vi "Compute Sum of Gates Plot.vi"(4 "SDV (s)":dbl=160.0, 6 "Gaussian IRF":bool, 8 "Error In":errorcluster, 10 "Phasor Parameters":T1={"Display Parameters"={"# Points"=0, "Ramp Type"=enum."Linear", "Type of Series"=enum."1-Exp Decays", "Min tau"=0.0, "Max tau"=0.0, "Include 0"=FALSE, "Include Infinity"=FALSE}, "Phasor Parameters"={"Harmonic frequency"=0.0, "Use f* = 1/D Frequency"=FALSE, "Calibrated Phasor"=FALSE, "Calibration Lifetime"=1e-09, "Phasor Calculation"=enum."Direct Sum", "SEPL Type"=enum."UC", "# Gates"=1.0, "Square Gate Width"=1e-09, "Show Ticks"=FALSE}, "Decay & IRF Parameters"={"Lifetime"=0.0, "IRF Offset"=0.0, "Laser Period"=0.0, "Normalized Decays"=FALSE, "IRF Model"=enum."Dirac", "IRF Parameter 1"=0.0}, "Gate Parameters"={"First Gate Start"=0.0, "Use Gate Center"=FALSE, "Gate Width"=0.0, "Gate Step"=0.0, "# Gates"=0.0, "Gate Type"=enum."Square", "Edge Width"=0.0, "Top Slope"=0.0, "Reversed Sawtooth?"=FALSE, "Analytical Computation"=FALSE, "Tolerance"=1.0, "Integration"=enum."Item 0", "# Steps"=1.0, "Type of User-defined Function"=enum."Gate"}, "Detector Parameters"={"Frames/Image"=0, "Gates/Frame"=0, "Bits/Frame"=0, "Multiplicity"=0, "Incident Signal"=0.0}} {"Detector Parameters"."Frames/Image" min=1; "Detector Parameters"."Multiplicity" min=0; "Detector Parameters"."Bits/Frame" min=1; "Detector Parameters"."Gates/Frame" min=1; "Gate Parameters"."# Steps" min=0.0; "Gate Parameters"."Tolerance" min=0.0; "Gate Parameters"."Top Slope" min=0.0; "Gate Parameters"."Edge Width" min=0.0; "Gate Parameters"."Gate Step" min=0.0; "Gate Parameters"."# Gates" min=0.0 step=1.0; "Gate Parameters"."Gate Width" min=0.0; "Decay & IRF Parameters"."Lifetime" min=0.0; "Decay & IRF Parameters"."Laser Period" min=0.0; "Phasor Parameters"."Square Gate Width" min=0.0; "Phasor Parameters"."# Gates" min=0.0; "Phasor Parameters"."Calibration Lifetime" min=0.0; "Phasor Parameters"."Harmonic frequency" min=0.0; "Display Parameters"."Min tau" min=0.0; "Display Parameters"."Max tau" min=0.0; "Display Parameters"."# Points" min=1 step=1}, 11 "Sum of Gates Graph Refnum":refnum<vi>) -> (0 "Error Out":errorcluster, 3 "Sum of Gates Plot":cluster{"Array":dbl[], "Array":dbl[]})   [LabVIEW 2019]
uses:
  Pseudo Phasor Parameters.ctl
  Phasor Explorer Display Parameters.ctl
  Type of Series.ctl
  Phasor Explorer Phasor Parameters.ctl
  Phasor Calculation Type.ctl
  Phasor Type.ctl
  Phasor Explorer Decay Parameters.ctl
  IRF Model.ctl
  Phasor Explorer Gate Parameters.ctl
  Gate Type.ctl
  Phasor Explorer Detector Parameters.ctl
  Linear Ramp End Options.ctl
  <vilib>/Utility/error.llb/Error Cluster From Error Code.vi
  SEPXP Globals.vi
  <vilib>/ErrorRing/Error Ring.xnode
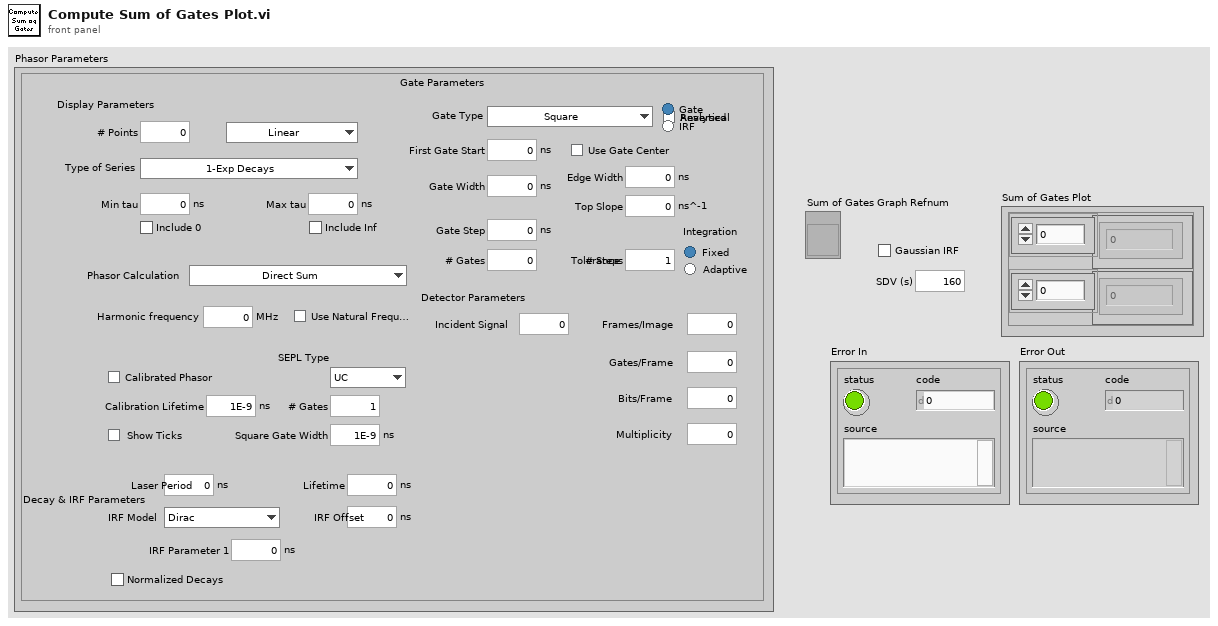
[diagram p1: front panel]
types:
  T1 = typedef "Pseudo Phasor Parameters.ctl" = cluster{"Display Parameters":T2, "Phasor Parameters":T4, "Decay & IRF Parameters":T7, "Gate Parameters":T9, "Detector Parameters":T11}
  T2 = typedef "Phasor Explorer Display Parameters.ctl" = cluster{"# Points":i32, "Ramp Type":enum16{"Linear", "Logarithmic"}, "Type of Series":T3, "Min tau":dbl[unit], "Max tau":dbl[unit], "Include 0":bool, "Include Infinity":bool}
  T3 = typedef "Type of Series.ctl" = enum16{"1-Exp Decays", "Linear Combination of 1-Exp"}
  T4 = typedef "Phasor Explorer Phasor Parameters.ctl" = cluster{"Harmonic frequency":dbl[unit], "Use f* = 1/D Frequency":bool, "Calibrated Phasor":bool, "Calibration Lifetime":dbl[unit], "Phasor Calculation":T5, "SEPL Type":T6, "# Gates":dbl, "Square Gate Width":dbl[unit], "Show Ticks":bool}
  T5 = typedef "Phasor Calculation Type.ctl" = enum16{"Direct Sum", "Analytical Formula"}
  T6 = typedef "Phasor Type.ctl" = enum16{"UC", "L_N", "L_N[W]"}
  T7 = typedef "Phasor Explorer Decay Parameters.ctl" = cluster{"Lifetime":dbl[unit], "IRF Offset":dbl[unit], "Laser Period":dbl[unit], "Normalized Decays":bool, "IRF Model":T8, "IRF Parameter 1":dbl[unit]}
  T8 = typedef "IRF Model.ctl" = enum16{"Dirac", "Exponential"}
  T9 = typedef "Phasor Explorer Gate Parameters.ctl" = cluster{"First Gate Start":dbl[unit], "Use Gate Center":bool, "Gate Width":dbl[unit], "Gate Step":dbl[unit], "# Gates":dbl, "Gate Type":T10, "Edge Width":dbl[unit], "Top Slope":dbl[unit], "Reversed Sawtooth?":bool, "Analytical Computation":bool, "Tolerance":dbl, "Integration":enum32{"Item 0", "Item 1"}, "# Steps":dbl, "Type of User-defined Function":enum32{"Gate", "IRF"}}
  T10 = typedef "Gate Type.ctl" = enum16{"Square", "Finite Edge Square", "Finite Edge, Tilted Top Square", "Triangle", "Sawtooth", "User-defined"}
  T11 = typedef "Phasor Explorer Detector Parameters.ctl" = cluster{"Frames/Image":i32, "Gates/Frame":i32, "Bits/Frame":i32, "Multiplicity":i32, "Incident Signal":dbl}
  T12 = typedef "Linear Ramp End Options.ctl" = enum16{"Include Min/Exclude Max", "Exclude Min/Include Max", "Include Both Ends", "Exclude Both Ends"}
  T13 = typedef "Gate Definitions.ctl" = cluster{"First Gate: t1":ext, "Gate Width: W":ext, "Gate Step: d":ext, "# Gates: G":ext, "Use Gate Center":bool, "Frames/Image: F":i32, "Gates/Frame: L":i32, "Bits/Frame: q":i32, "Multiplicity: p":i32, "Gate Type":T10, "Gate Edge s":ext, "Gate Top Slope":ext, "Reversed Sawtooth?":bool, "Computation":bool, "User-defined Gate":T14, "Tolerance":ext, "Integration":enum32{"Item 0", "Item 1"}, "# Steps":ext, "Type of User-defined Function":enum32{"Gate", "IRF"}}
  T14 = typedef "XY Plot Data.ctl" = cluster{"X Array":dbl[], "Y Array":dbl[]}
  T15 = typedef "Decay Definiton.ctl" = cluster{"offset: t0":ext, "period: T":ext, "lifetime: tau":ext, "Incident Signal: I":ext, "Normalized Decays":bool, "IRF Model":T8, "IRF Parameter 1":ext}
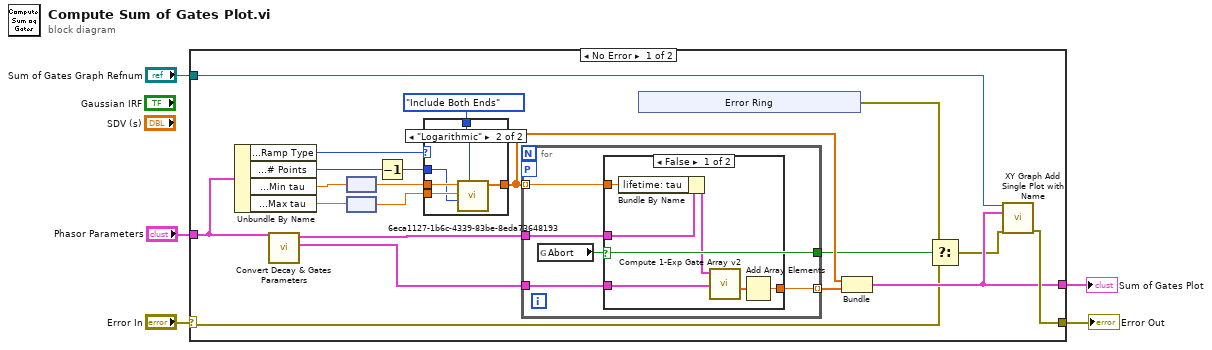
[diagram p0: block diagram]
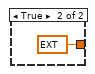
[diagram p2: hidden frame]
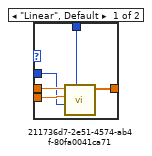
[diagram p3: hidden frame]
diagram:
  n1 = case shown="No Error" "Error In" {
    selector: "Error In" -> [w8 w52]
    tunnel: "Phasor Parameters" -> [w13 _]
    tunnel: "Sum of Gates Graph Refnum" -> [w21 _]
    tunnel: [w20 w52] -> w2
    tunnel: [w14 _] -> w1
    frame No Error {
      n2 = Unbundle By Name(w13) -> ("Display Parameters.Ramp Type"=w19:enum16{"Linear", "Logarithmic"}, "Display Parameters.# Points"=w16:i32, "Display Parameters.Min tau"=w24:dbl[unit], "Display Parameters.Max tau"=w25:dbl[unit])
      n3 = call "Convert Decay & Gates Parameters.vi"("Phasor Parameters"=w13) -> ("Gates Definitions"=w11:T13, "Decay Definition"=w12:T15)  [unwired: 9 in]
      n4 = node(w24) -> (w23:dbl)
      n5 = node(w25) -> (w22:dbl)
      n6 = Decrement(x=w16) -> (x-1=w17:i32)
      n7 = case shown="\"Logarithmic\"" w19 {
        tunnel: w23 -> [w46 w49]
        tunnel: w22 -> [w45 w48]
        tunnel: w17 -> [w44 w47]
        tunnel: [w43 w51] -> w10
        tunnel: Linear_Ramp_End_Options."Include Both Ends" ("Options") -> [w42 w50]
        frame "Linear", Default {
          n8 = call "211736d7-2e51-4574-ab4f-80fa0041ca71.vi"("Options"=w42, "# Steps (1)"=w44, "End (1)"=w45, "Start (0)"=w46) -> ("Ramp"=w43:dbl[])  [unwired: 6 in, 1 out]
        }
        frame "Logarithmic" {
          n9 = call "6eca1127-1b6c-4339-83be-8eda73648193.vi"("Options"=w50, "# Steps (1)"=w47, "End (1)"=w48, "Start (1)"=w49) -> ("Ramp"=w51:dbl[])  [unwired: 6 in, 1 out]
        }
      }
      n10 = for {
        tunnel: w10 -> [w34] mode=indexing
        tunnel: w11 -> [w32]
        tunnel: w12 -> [w33]
        tunnel: [w31] -> w15 mode=indexing
        workers-P: _ -> [_]
        tunnel: [w30] -> w9
        n11 = global read "SEPXP Globals.vi" "Abort"() -> (w30:bool)
        n12 = case shown="False" w30 {
          tunnel: w34 -> [w40 _]
          tunnel: w33 -> [w39 _]
          tunnel: w32 -> [w37 _]
          tunnel: [w35 ext nan ("Numeric Control")] -> w31
          frame False {
            n13 = Bundle By Name(cluster=w39, "lifetime: tau"=w40) -> (w38:T15)
            n14 = call "Compute 1-Exp Gate Array v2.vi"("Gates Definitions"=w37, "Decay Definition"=w38) -> ("Gate Image Array"=w36:ext[])  [unwired: 5 in, 4 out]
            n15 = Add Array Elements(numeric array=w36) -> (sum=w35:ext)
          }
          frame True {
          }
        }
      }
      n16 = xnode "Error Ring"() -> ("error out"=w6:errorcluster)
      n17 = Bundle("Ramp"=w10, w15) -> (w14:cluster{"Ramp":dbl[], ext[]})  [unwired: 1 in]
      n18 = Select(t=w6, s=w9, f=w8) -> (s? t:f=w7:errorcluster)
      n19 = call "XY Graph Add Single Plot with Name.vi"("XYGraph Ref in"=w21, "Plot"=w14, "error in (no error)"=w7) -> ("error out"=w20:errorcluster)  [unwired: 9 in, 3 out]
    }
    frame Error {
    }
  }
  "Error Out" <- w2
  "Sum of Gates Plot" <- w1
